vi "WCA_set_PLL_para.vi"(0 "ObjHandle in":u32, 2 "LO_FREQ_SET":T1={"YTO Low freq. [GHz]"=12.17, "YTO High freq. [GHz]"=14.833, "Kvco"=1, "Lock Pol."=0, "SET LO FREQ"=25.0, "Multiplier"=3.0, "YTO coarse tune(HEX)"=0, "YTO coarse( FREQ)"=25.0, "NULL PLL INTEGRATOR"=FALSE} {"YTO coarse( FREQ)" min=25 max=150 step=0.0001 format="%.3f"; "YTO coarse tune(HEX)" format="%x"; "Multiplier" min=3 max=6 step=3; "SET LO FREQ" min=25 max=150 step=0.0001 format="%.3f"; "Lock Pol." items=["Lower", "Upper"]; "Kvco" items=["7.5MHz/V", "15MHz/V"]; "YTO High freq. [GHz]" format="%.3f"; "YTO Low freq. [GHz]" format="%.3f"}, 5 "error in (no error)":errorcluster, 10 "Slave Node in":cluster{"Address":i16, "Serial Number":i8[]}={"Address"=19, "Serial Number"=[16, 71, 55, 76, 1, 8, 0, -15]} {"Serial Number" format="%.0x"; "Address" format="%.0x"}, 12 "Cartridge band":u32 max=10 step=1) -> (16 "LO_FREQ_SET output":T1={"YTO Low freq. [GHz]"=12.17, "YTO High freq. [GHz]"=14.833, "Kvco"=1, "Lock Pol."=0, "SET LO FREQ"=25.0, "Multiplier"=3.0, "YTO coarse tune(HEX)"=0, "YTO coarse( FREQ)"=25.0, "NULL PLL INTEGRATOR"=FALSE} {"YTO coarse( FREQ)" min=25 max=150 step=0.0001 format="%.3f"; "YTO coarse tune(HEX)" format="%x"; "Multiplier" min=3 max=6 step=3; "SET LO FREQ" min=25 max=150 step=0.0001 format="%.3f"; "Lock Pol." items=["Lower", "Upper"]; "Kvco" items=["7.5MHz/V", "15MHz/V"]; "YTO High freq. [GHz]" format="%.3f"; "YTO Low freq. [GHz]" format="%.3f"}, 19 "error out":errorcluster)   [LabVIEW 2017]
panel:
  out "YTOSet":u16
  out "ObjHandle out":u32
  # "LO freq. [GHz]"
  # "ZERO Intgrtr"
  # "LO freq. [GHz]"
  # "ZERO Intgrtr"
  # "Node Address"
  # "Serial Number"
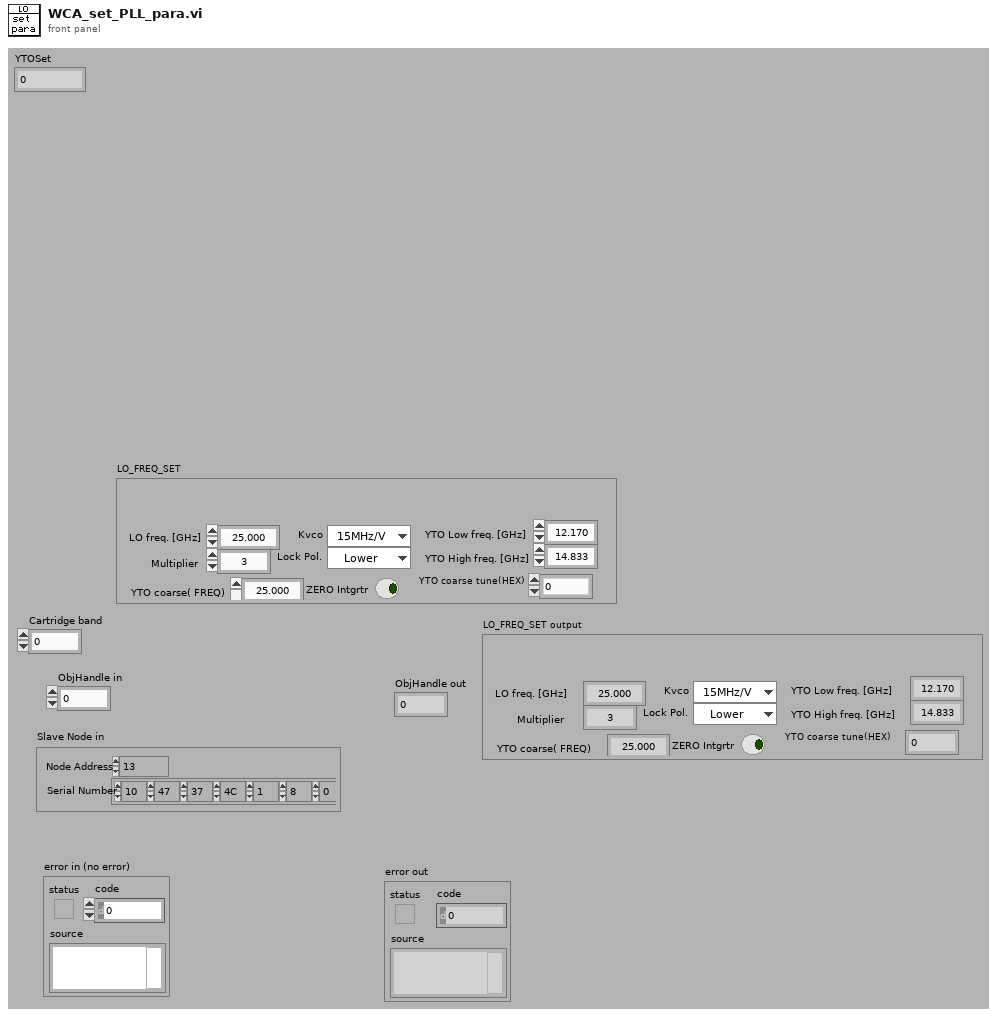
[diagram p1: front panel]
types:
  T1 = cluster{"YTO Low freq. [GHz]":sgl, "YTO High freq. [GHz]":sgl, "Kvco":u16, "Lock Pol.":u16, "SET LO FREQ":sgl, "Multiplier":sgl, "YTO coarse tune(HEX)":u16, "YTO coarse( FREQ)":sgl, "NULL PLL INTEGRATOR":bool}
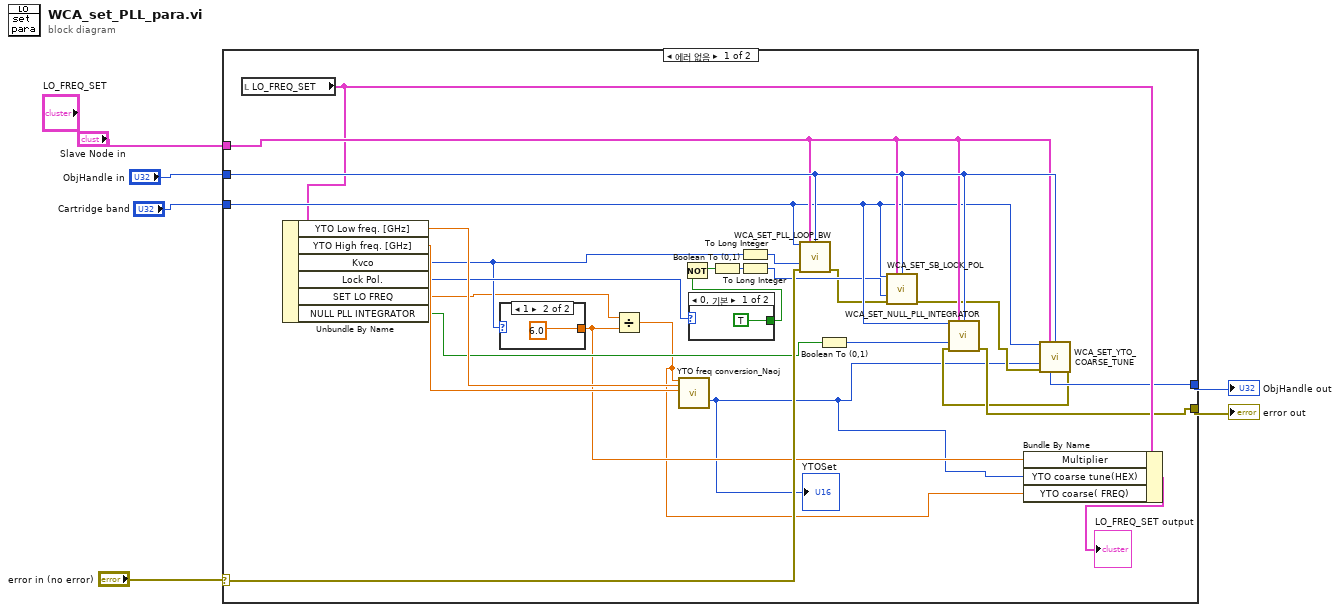
[diagram p0: block diagram]
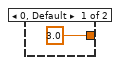
[diagram p2: hidden frame]
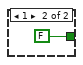
[diagram p3: hidden frame]
diagram:
  n1 = case shown="에러 없음" "error in (no error)" {
    selector: "error in (no error)" -> [w32 w38]
    tunnel: "ObjHandle in" -> [w31 w37]
    tunnel: "Slave Node in" -> [w30 _]
    tunnel: [w13 w37] -> w1
    tunnel: [w12 w38] -> w4
    tunnel: "Cartridge band" -> [w29 _]
    frame No Error {
      n2 = local read "LO_FREQ_SET"() -> (w15:T1)
      n3 = Unbundle By Name(w15) -> ("YTO Low freq. [GHz]"=w24:sgl, "YTO High freq. [GHz]"=w23:sgl, "Kvco"=w18:u16, "Lock Pol."=w22:u16, "SET LO FREQ"=w17:sgl, "NULL PLL INTEGRATOR"=w19:bool)
      n4 = case shown="1" w18 {
        tunnel: [sgl 3.0 sgl 6.0] -> w16
        frame 0, Default {
        }
        frame 1 {
        }
      }
      n5 = Divide(x=w17, y=w16) -> (x/y=w7:sgl)
      n6 = call "YTO freq conversion_Naoj.vi"("YTO desired frequency"=w7, "YTO freq Min"=w24, "YTO freq. Max"=w23) -> ("YTO Coarse tune"=w8:u16)  [unwired: 16 in]
      "YTOSet" <- w8
      n7 = case shown="0, 기본" w22 {
        tunnel: [TRUE FALSE] -> w21
        frame 0, Default {
        }
        frame 1 {
        }
      }
      n8 = Not(x=w21) -> (.not. x?=w9:bool)
      n9 = Boolean To (0,1)(Boolean=w9) -> (0, 1=w28:i16)
      n10 = To Long Integer(number=w18) -> (32bit integer=w27:i32)
      n11 = To Long Integer(number=w28) -> (32bit integer=w26:i32)
      n12 = call "WCA_SET_PLL_LOOP_BW.vi"("Cartridge Band"=w29, "Slave Node in"=w30, "ObjHandle in"=w31, "SET_PLL_LOOP_BW"=w27, "error in (no error)"=w32) -> ("error out"=w25:errorcluster)  [unwired: 9 in, 1 out]
      n13 = Boolean To (0,1)(Boolean=w19) -> (0, 1=w20:i16)
      n14 = call "WCA_SET_SB_LOCK_POL.vi"("Cartridge Band"=w29, "Slave Node in"=w30, "ObjHandle in"=w31, "SET_SB_LOCK_POL"=w26, "error in (no error)"=w25) -> ("error out"=w11:errorcluster)  [unwired: 9 in, 1 out]
      n15 = Bundle By Name(cluster=w15, "Multiplier"=w16, "YTO coarse tune(HEX)"=w8, "YTO coarse( FREQ)"=w7) -> (→"LO_FREQ_SET output":T1)
      n16 = call "WCA_SET_YTO_COARSE_TUNE.vi"("Cartridge Band"=w29, "Slave Node in"=w30, "ObjHandle in"=w31, "SET_YTO_COARSE_TUNE"=w8, "error in (no error)"=w11) -> ("ObjHandle out"=w13:u32, "error out"=w10:errorcluster)  [unwired: 9 in]
      n17 = call "WCA_SET_NULL_PLL_INTEGRATOR.vi"("Cartridge Band"=w29, "Slave Node in"=w30, "ObjHandle in"=w31, "SET_NULL_PLL_INTEGRATOR"=w20, "error in (no error)"=w10) -> ("error out"=w12:errorcluster)  [unwired: 9 in, 1 out]
    }
    frame Error {
      (unwired) sgl -1.0 ("SET YTO COARSE TUNE")
    }
  }
  "error out" <- w4
  "ObjHandle out" <- w1
